vi "round.step.4.5.6.7.vi"(9 "D.in":u64[](array[numeric]), 10 "state[25]":u64[](array[numeric]), 11 "Parameters":T1[](array[typedef])=[{"Left_Shift"=1, "State_Index"=1, "D_Index"=1}, {"Left_Shift"=6, "State_Index"=7, "D_Index"=2}, {"Left_Shift"=25, "State_Index"=13, "D_Index"=3}, {"Left_Shift"=8, "State_Index"=19, "D_Index"=4}, {"Left_Shift"=18, "State_Index"=20, "D_Index"=0}]) -> (2 "E.out":u64[](array[numeric]) format="%.0x", 3 "B.out":u64[](array[numeric]) format="%.0x")   [LabVIEW 2021]
uses:
  Step.4.5.6.7.Inputs.ctl
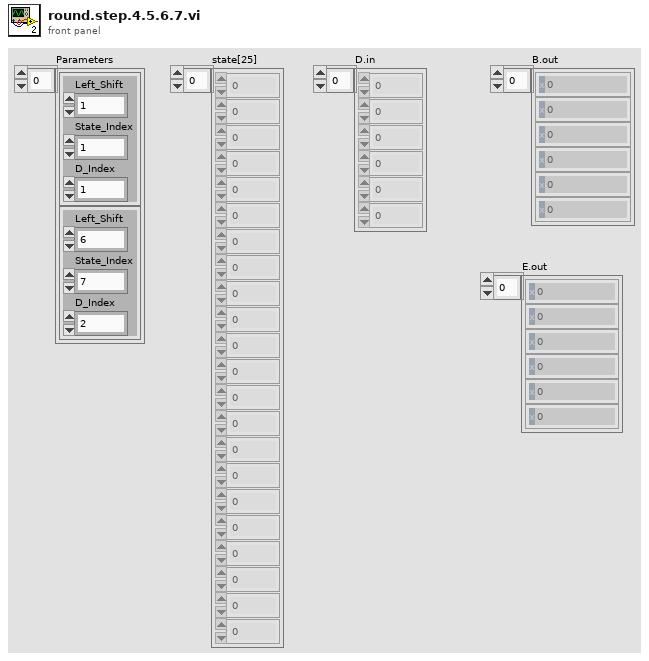
[diagram p1: front panel]
types:
  T1 = typedef "Step.4.5.6.7.Inputs.ctl" = cluster{"Left_Shift":i32, "State_Index":i32, "D_Index":i32}
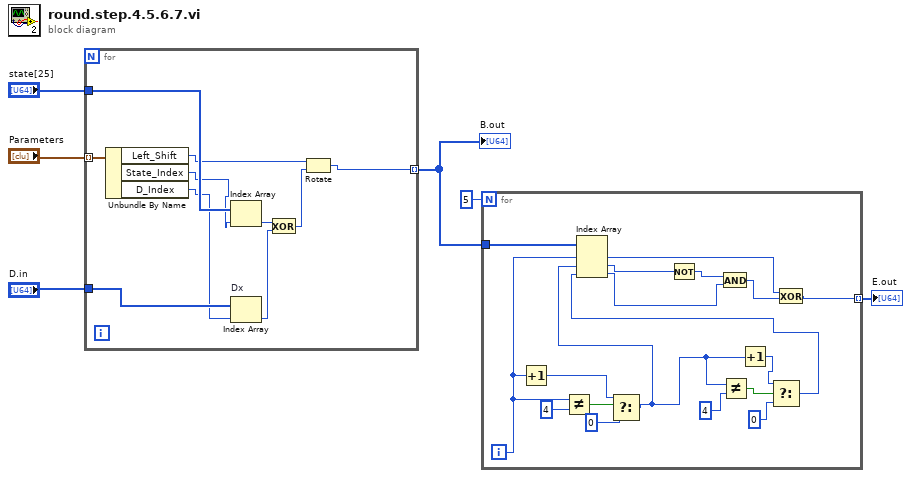
[diagram p0: block diagram]
diagram:
  n1 = for {
    tunnel: "Parameters" -> [w16] mode=indexing
    tunnel: "D.in" -> [w12]
    tunnel: "state[25]" -> [w11]
    tunnel: [w7] -> w3 mode=indexing
    n2 = Unbundle By Name(w16) -> ("Left_Shift"=w9:i32, "State_Index"=w8:i32, "D_Index"=w10:i32)
    n3 = Index Array(array=w11, index=w8) -> (element=w15:u64)
    n4 = Index Array "Dx"(array=w12, index=w10) -> (element=w13:u64)
    n5 = Exclusive Or(1:w13, 2:w15) -> (0:w14:u64)
    n6 = Rotate(1:w14, 2:w9) -> (0:w7:u64)
  }
  "B.out" <- w3
  n7 = for {
    N: 5 -> [_]
    tunnel: w3 -> [w34]
    tunnel: [w28] -> w1 mode=indexing
    i -> [w27]
    n8 = Increment(x=w27) -> (x+1=w23:i32)
    n9 = Not Equal?(x=w27, y=4) -> (x != y?=w25:bool)
    n10 = Select(t=w23, s=w25, f=0) -> (s? t:f=w22:i32)
    n11 = Not Equal?(x=w22, y=4) -> (x != y?=w20:bool)
    n12 = Increment(x=w22) -> (x+1=w19:i32)
    n13 = Select(t=w19, s=w20, f=0) -> (s? t:f=w18:i32)
    n14 = Index Array(array=w34, index #1=w27, index #2=w22, index #3=w18) -> (element #1=w29:u64, element #2=w32:u64, element #3=w31:u64)
    n15 = Not(x=w32) -> (.not. x?=w33:u64)
    n16 = And(x=w33, y=w31) -> (x .and. y?=w30:u64)
    n17 = Exclusive Or(1:w30, 2:w29) -> (0:w28:u64)
  }
  "E.out" <- w1
